vi "Test make file names.vi"() -> ()   [LabVIEW 2015]
uses:
  Controls/File formats.ctl
panel:
  out "Settings File Path":path
  out "Data File  Path":path
  in  "File Prefix":string="rt"
  in  "Root Data Folder":path=path "D:/Data"
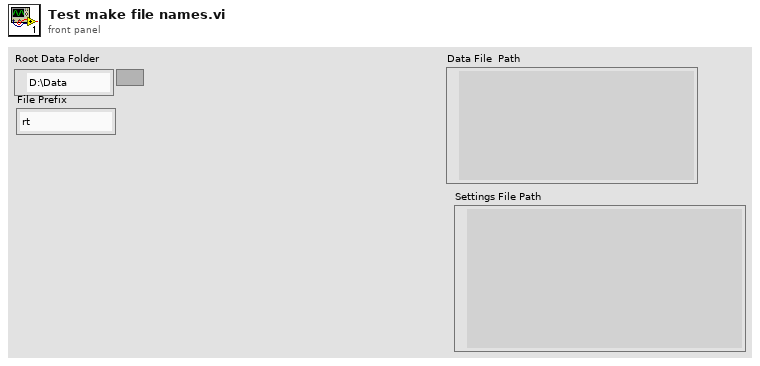
[diagram p1: front panel]
types:
  T1 = typedef "File formats.ctl" = enum16{"TDMS", "ASCII", "BINARY"}
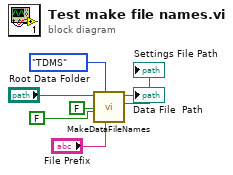
[diagram p0: block diagram]
diagram:
  n1 = call "MakeDataFileNames.vi"("File Prefix"="File Prefix", "File format"=File_formats."TDMS", "Interactive"=FALSE ("Generate Index"), "Generate Index"=FALSE, "Root Data Folder"="Root Data Folder") -> ("Settings File Path"=→"Settings File Path":path, "Data File  Path"=→"Data File  Path":path)  [unwired: 4 in, 1 out]
